vi "Configure DC Current.vi"(5 "NPLC":dbl=1.0, 6 "Aperture Seconds":dbl, 7 "Set Aperture or NPLC":bool=TRUE, 8 "error in (no error)":errorcluster, 9 "Manual Range":dbl=3.0, 10 "Auto Range? (T: Auto)":bool, 11 "VISA resource name":refnum<visa-resource-name>) -> (0 "error out":errorcluster, 3 "VISA resource name out":refnum<visa-resource-name>)   [LabVIEW 2025, in "Keithley DMM7510.lvlib"]
doc: "This VI configures the DC Current measurement and the related parameters."
uses:
  Keithley DMM7510.lvlib
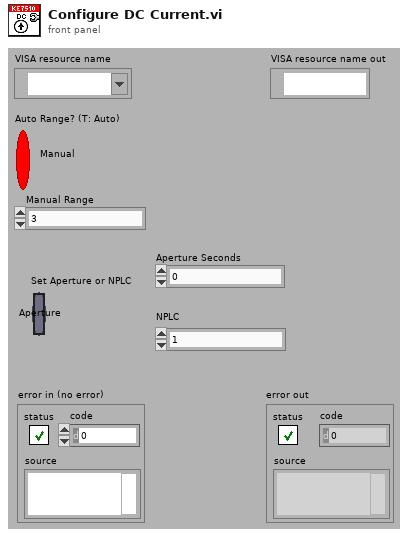
[diagram p1: front panel]
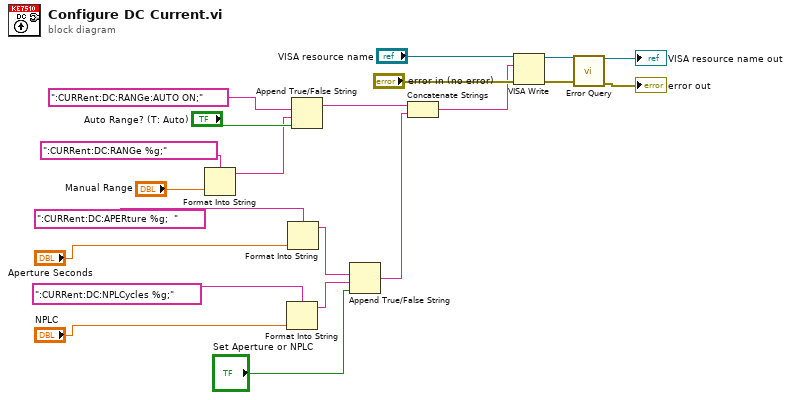
[diagram p0: block diagram]
diagram:
  n1 = Format Into String(format string=":CURRent:DC:RANGe %g;", "Manual Range") -> (resulting string=w15:string)  [unwired: 2 in, 1 out]
  n2 = Format Into String(format string=":CURRent:DC:NPLCycles %g;", "NPLC") -> (resulting string=w3:string)  [unwired: 2 in, 1 out]
  n3 = Format Into String(format string=":CURRent:DC:APERture %g;  ", "Aperture Seconds") -> (resulting string=w2:string)  [unwired: 2 in, 1 out]
  n4 = Append True/False String(1:"Auto Range? (T: Auto)", 2:w15, 3:":CURRent:DC:RANGe:AUTO ON;") -> (0:w12:string)  [unwired: 1 in]
  n5 = Append True/False String(1:"Set Aperture or NPLC", 2:w3, 3:w2) -> (0:w1:string)  [unwired: 1 in]
  n6 = Concatenate Strings(w12, w1) -> (w11:string)
  n7 = VISA Write(VISA resource name="VISA resource name", write buffer=w11, error in (no error)="error in (no error)") -> (VISA resource name out=w10:refnum<visa-resource-name>, error out=w9:errorcluster)  [unwired: 1 out]
  n8 = call "Error Query.vi"("error in (no error)"=w9, "VISA resource name"=w10) -> ("error out"=→"error out":errorcluster, "VISA resource name out"=→"VISA resource name out":refnum<visa-resource-name>)  [unwired: 6 in, 2 out]
